vi "Find Measurement Monitoring Service.vi"() -> ()   [LabVIEW 2023]
uses:
  <vilib>/MeasurementLink/MeasurementLink Discovery Client/RPC Messages/ni_measurementlink_discovery_v1_ServiceLocation.ctl
  Measurement Configuration.ctl
  <vilib>/MeasurementLink/MeasurementLink Discovery Client/RPC Messages/ni_measurementlink_discovery_v1_EnumerateServicesRequest.ctl
  <vilib>/MeasurementLink/MeasurementLink Discovery Client/RPC Messages/ni_measurementlink_discovery_v1_ResolveServiceRequest.ctl
  Measurement Results.ctl
  MeasurementLink measurement_client/RPC Messages/ni_measurementlink_measurement_v1_MeasureRequest.ctl
  MeasurementLink measurement_client/RPC Messages/google_protobuf_Any.ctl
  MeasurementLink measurement_client/RPC Messages/ni_measurementlink_PinMapContext.ctl
  5395de1c-0486-4efa-930b-a2691ac7744a.vi
  <vilib>/gRPC/LabVIEW gRPC Library/Server API/Translate Protobuf Error.vi
  <vilib>/AdvancedString/1D String Array to Delimited String.vi
  <vilib>/gRPC/LabVIEW gRPC Library/Server API/Server/Get Server DLL Path.vi
  <vilib>/MeasurementLink/MeasurementLink Discovery Client/MeasurementLink Discovery Client.lvlib
  <vilib>/gRPC/LabVIEW gRPC Library/grpc-lvsupport-release.lvlib
  MeasurementLink measurement_client/MeasurementLink measurement_client.lvlib
  monitoring_metadata_client/monitoring_metadata_client.lvlib
panel:
  out "Waveform Graph":dbl[](graph)
  in  "Measurement Configuration":T1={"Frequency"=1, "Amplitude"=1}
  out "Available Services":string[](array[string])
  out "error out":errorcluster
  out "Matched Service":T2
  out "Found?":bool
  in  "address":string="localhost:42000"
  in  "Service To find":string="MyFirstPythonMeas_Python"
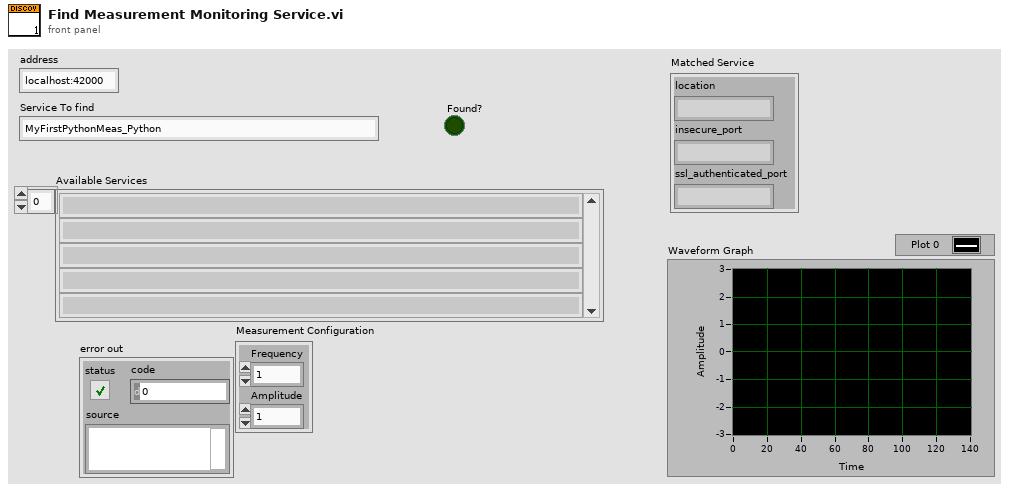
[diagram p1: front panel]
types:
  T1 = typedef "Measurement Configuration.ctl" = cluster{"Frequency":u32, "Amplitude":u32}
  T2 = typedef "MeasurementLink Discovery Client.lvlib/ni_measurementlink_discovery_v1_ServiceLocation.ctl" = cluster{"location":string, "insecure_port":string, "ssl_authenticated_port":string}
  T3 = typedef "Measurement Results.ctl" = cluster{"Array":dbl[]}
  T4 = typedef "MeasurementLink Discovery Client.lvlib/ni_measurementlink_discovery_v1_ResolveServiceRequest.ctl" = cluster{"provided_interface":string, "service_class":string}
  T5 = typedef "MeasurementLink Discovery Client.lvlib/ni_measurementlink_discovery_v1_EnumerateServicesRequest.ctl" = cluster{"provided_interface":string}
  T6 = typedef "grpc-lvsupport-release.lvlib/grpcId.ctl" = u64
  T7 = typedef "MeasurementLink Discovery Client.lvlib/ni_measurementlink_discovery_v1_EnumerateServicesResponse.ctl" = cluster{"available_services":T8[]}
  T8 = typedef "MeasurementLink Discovery Client.lvlib/ni_measurementlink_discovery_v1_ServiceDescriptor.ctl" = cluster{"display_name":string, "description_url":string, "provided_interfaces":string[], "service_class":string, "annotations":T9[]}
  T9 = typedef "MeasurementLink Discovery Client.lvlib/ni_measurementlink_discovery_v1_ServiceDescriptor_AnnotationsEntry.ctl" = cluster{"key":string, "value":string}
  T10 = typedef "grpc-lvsupport-release.lvlib/Message Metadata.ctl" = cluster{"Version":i32, "Name":string, "Type Url":string, "Elements":T11[]}
  T11 = typedef "grpc-lvsupport-release.lvlib/Message Element Metadata.ctl" = cluster{"Embedded Message Name":string, "Protobuf Index":i32, "MessageElementType":T12, "Repeated":bool}
  T12 = typedef "grpc-lvsupport-release.lvlib/Message Element Type.ctl" = enum32{"Int32Value", "FloatValue", "DoubleValue", "BoolValue", "StringValue", "MessageValue", "Int64Value", "UInt32Value", "UInt64Value", "EnumValue", "Bytes", "Fixed64", "Fixed32", "SFixed64", "SFixed32", "SInt64", "SInt32"}
  T13 = typedef "MeasurementLink measurement_client.lvlib/ni_measurementlink_measurement_v1_MeasureRequest.ctl" = cluster{"configuration_parameters":T14, "pin_map_context":T15}
  T14 = typedef "MeasurementLink measurement_client.lvlib/google_protobuf_Any.ctl" = cluster{"type_url":string, "value":u8[]}
  T15 = typedef "MeasurementLink measurement_client.lvlib/ni_measurementlink_PinMapContext.ctl" = cluster{"pin_map_id":string, "sites":i32[]}
  T16 = typedef "grpc-lvsupport-release.lvlib/Any.ctl" = cluster{"Type Url":string, "Bytes":u8[]}
  T17 = typedef "MeasurementLink measurement_client.lvlib/ni_measurementlink_measurement_v1_MeasureResponse.ctl" = cluster{"outputs":T14}
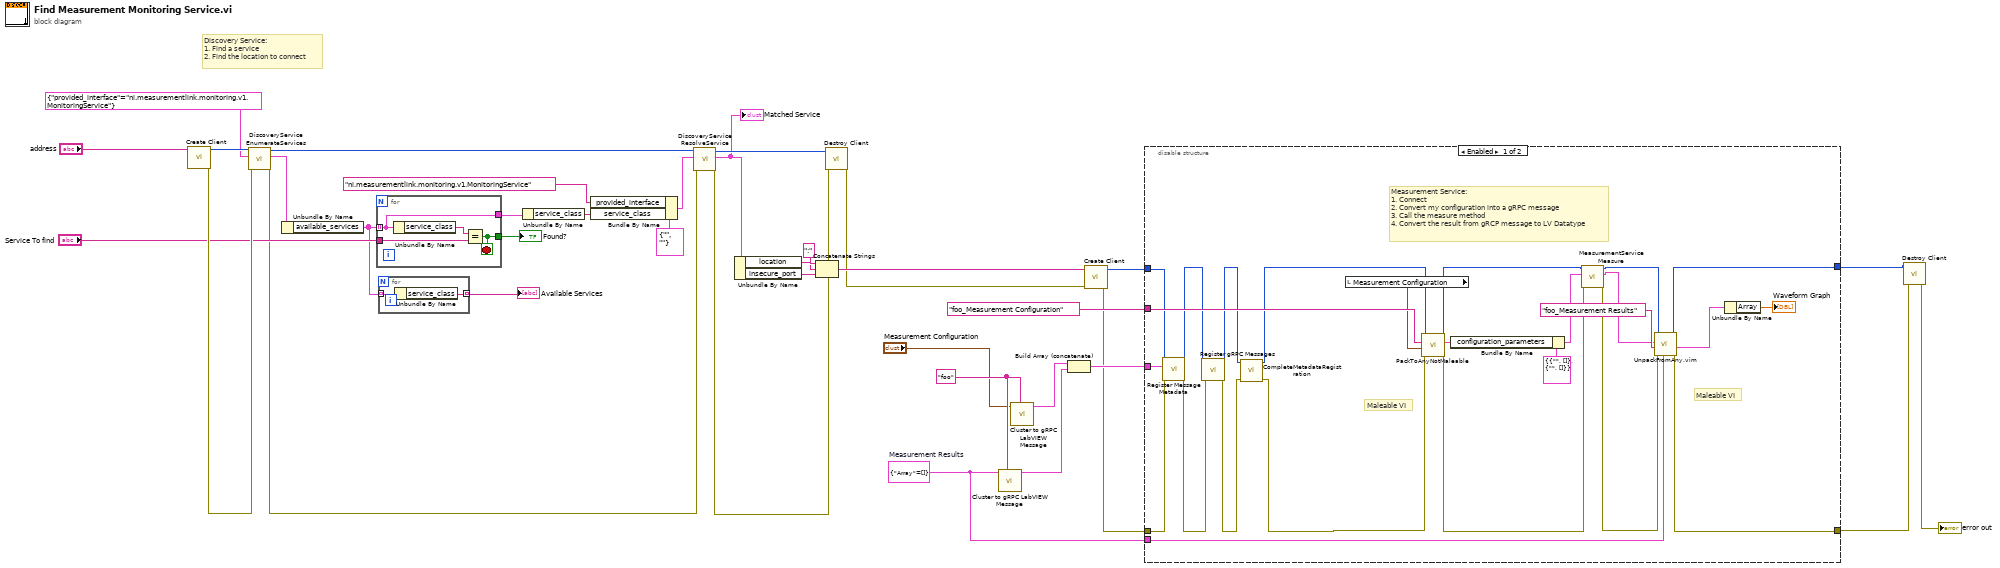
[diagram p0: block diagram]
diagram:
  w5 = T3 {"Array"=[]}  # Measurement Results
  w13 = "foo" ("Package Name")
  # "Discovery Service:\n1. Find a service\n2. Find the location to connect"
  n1 = call <vilib>:"Create Client.vi"("address"="address") -> ("error out"=w34:errorcluster, "gRPC ID Out"=w35:T6)  [unwired: 9 in]
  n2 = call <vilib>:"DiscoveryService EnumerateServices.vi"("error in"=w34, "Request Data"=T5 {"provided_interface"="ni.measurementlink.monitoring.v1.MonitoringService"}, "gRPC ID"=w35) -> ("error out"=w27:errorcluster, "Response Data"=w32:T7, "gRPC ID out"=w28:T6)  [unwired: 6 in]
  n3 = Unbundle By Name(w32) -> ("available_services"=w20:T8[])
  n4 = for {
    tunnel: w20 -> [w38] mode=indexing
    tunnel: "Service To find" -> [w39]
    tunnel: [w38] -> w29
    tunnel: [w37] -> w30
    stop <- w37 stop-if-true
    n5 = Unbundle By Name(w38) -> ("service_class"=w40:string)
    n6 = Equal?(x=w40, y=w39) -> (x = y?=w37:bool)
  }
  "Found?" <- w30
  n7 = for {
    tunnel: w20 -> [w42] mode=indexing
    tunnel: [w41] -> w19 mode=indexing
    n8 = Unbundle By Name(w42) -> ("service_class"=w41:string)
  }
  "Available Services" <- w19
  n9 = Unbundle By Name(w29) -> ("service_class"=w23:string)
  n10 = Bundle By Name(cluster=T4 {"provided_interface"="", "service_class"=""} ("Request Data"), "provided_interface"="ni.measurementlink.monitoring.v1.MonitoringService", "service_class"=w23) -> (w21:T4)
  n11 = call <vilib>:"DiscoveryService ResolveService.vi"("error in"=w27, "Request Data"=w21, "gRPC ID"=w28) -> ("error out"=w26:errorcluster, "Response Data"=w3:T2, "gRPC ID out"=w25:T6)  [unwired: 6 in]
  "Matched Service" <- w3
  n12 = Unbundle By Name(w3) -> ("location"=w18:string, "insecure_port"=w16:string)
  n13 = Concatenate Strings(w18, ":" ("string"), w16) -> (w10:string)
  n14 = call <vilib>:"Destroy Client.vi"("error in"=w26, "gRPC ID"=w25) -> ("error out"=w2:errorcluster)  [unwired: 9 in]
  n15 = call <vilib>:"Cluster to gRPC LabVIEW Message.vi"("Package Name"=w13, "Cluster"=w5) -> ("gRPC Message Metadata []"=w14:T10[])  [unwired: 8 in, 1 out]
  n16 = call <vilib>:"Cluster to gRPC LabVIEW Message.vi"("Package Name"=w13, "Cluster"="Measurement Configuration") -> ("gRPC Message Metadata []"=w15:T10[])  [unwired: 8 in, 1 out]
  n17 = Build Array (concatenate)(w15, w14) -> (w12:T10[])
  n18 = call <vilib>:"Create Client.vi"("error in"=w2, "address"=w10) -> ("error out"=w9:errorcluster, "gRPC ID Out"=w8:T6)  [unwired: 8 in]
  n19 = disable-structure shown="Enabled" {
    disable-tunnel: w12 -> [w67 _]
    disable-tunnel: "foo_Measurement Configuration" ("Message Type") -> [w66 _]
    disable-tunnel: w9 -> [w65 w68]
    disable-tunnel: w8 -> [w64 w69]
    disable-tunnel: [w63 w69] -> w7
    disable-tunnel: [w62 w68] -> w6
    disable-tunnel: w5 -> [w61 _]
    frame Enabled {
      # "Maleable VI"
      # "Maleable VI"
      # "Measurement Service:\n1. Connect\n2. Convert my configuration into a gRPC message\n3. Call the measure method\n4. Convert the result from gRCP message to LV Datatype"
      n20 = call <vilib>:"Register Message Metadata.vi"("error in"=w65, "Messages"=w67, "gRPCid in"=w64) -> ("error out"=w44:errorcluster, "gRPCid out"=w46:T6)  [unwired: 7 in]
      n21 = call "Register gRPC Messages.vi"("error in (no error)"=w44, "gRPC ID"=w46) -> ("error out"=w43:errorcluster, "gRPC ID Out"=w45:T6)  [unwired: 8 in]
      n22 = call <vilib>:"CompleteMetadataRegistration.vi"("error in"=w43, "gRPC ID in"=w45) -> ("error out"=w59:errorcluster, "gRPC ID Out"=w60:T6)  [unwired: 8 in]
      n23 = local read "Measurement Configuration"() -> (w49:T1)
      n24 = call "PackToAnyNotMaleable.vi"("error in"=w59, "Data To Pack"=w49, "Message Type"=w66, "gRPCid in"=w60) -> ("error out"=w48:errorcluster, "Any"=w47:T16, "gRPCid out"=w57:u64)  [unwired: 5 in]
      n25 = Bundle By Name(cluster=T13 {"configuration_parameters"={"type_url"="", "value"=[]}, "pin_map_context"={"pin_map_id"="", "sites"=[]}} ("Request Data"), "configuration_parameters"=w47) -> (w53:T13)
      n26 = call "MeasurementService Measure.vi"("error in"=w48, "Request Data"=w53, "gRPC ID"=w57) -> ("error out"=w55:errorcluster, "Response Data"=w50:T17, "gRPC ID out"=w56:T6)  [unwired: 6 in]
      n27 = call "UnpackFromAny.vim"("Data Type"=w61, "error in"=w55, "Message Type"="foo_Measurement Results", "Any"=w50, "gRPCid in"=w56) -> ("error out"=w62:errorcluster, "Unpacked Value"=w51:T3, "gRPCid out"=w63:u64)  [unwired: 4 in]
      n28 = Unbundle By Name(w51) -> ("Array"=→"Waveform Graph":dbl[])
    }
    frame Disabled {
    }
  }
  n29 = call <vilib>:"Destroy Client.vi"("error in"=w6, "gRPC ID"=w7) -> ("error out"=→"error out":errorcluster)  [unwired: 9 in]
